vi "To Waveform.vi"(8 "error in (no error)":errorcluster, 11 "I32 in":refnum<class "I32.lvclass">) -> (0 "error out":errorcluster, 1 "Success?":bool, 3 "Waveform Array":waveform(dbl)[](array[waveform]))   [LabVIEW 2020, in "Data.lvlib" / "I32.lvclass"]
doc: "Interpret 'Data' as a Waveform Array. If impossible 'Success?' is set to FALSE"
uses:
  I32.lvclass
  I32.lvclass/I32.ctl
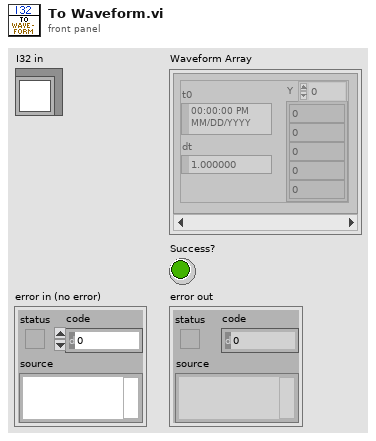
[diagram p1: front panel]
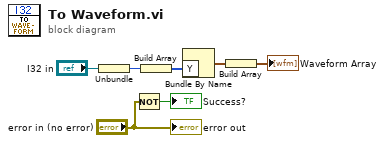
[diagram p0: block diagram]
diagram:
  n1 = Unbundle("I32 in") -> (w6:i32)
  n2 = Not(x="error in (no error)") -> (.not. x?=→"Success?":bool)
  n3 = Build Array(w6) -> (w4:i32[])
  n4 = Bundle By Name("Y"=w4) -> (w7:waveform(i32))  [unwired: 1 in]
  n5 = Build Array(w7) -> (→"Waveform Array":waveform(i32)[])
  "error out" <- "error in (no error)"
